vi "DB Info.vi"(8 "error in (no error)":errorcluster, 11 "Access in":refnum<class "Access.lvclass">) -> (0 "error out":errorcluster, 1 "Column_info":T1, 2 "Table_info":T4, 3 "Access out":refnum<class "Access.lvclass">)   [LabVIEW 2021, in "Database.lvlib" / "Access.lvclass"]
uses:
  Access.lvclass
  DB/Table_info.ctl
  DB/Column_info.ctl
  <vilib>/addons/database/Auxilliary.llb/DB Tools Column Info.ctl
  <vilib>/addons/database/Auxilliary.llb/DB Tools DataTypes.ctl
  DB/DB.lvclass
  <vilib>/addons/database/NI_Database_API.lvlib
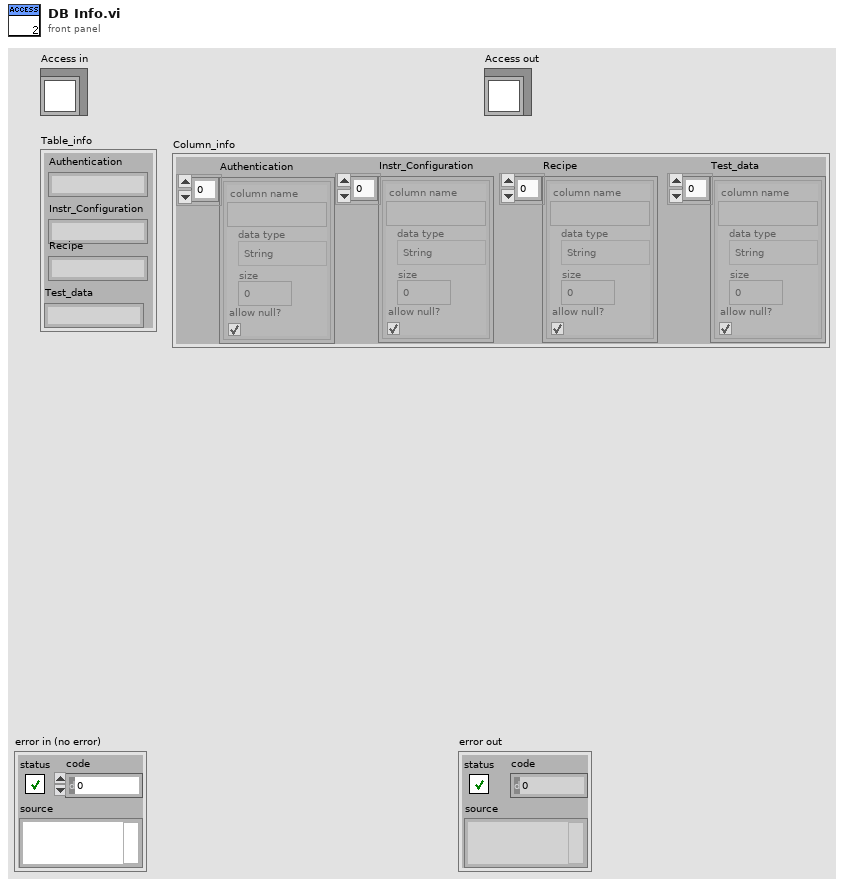
[diagram p1: front panel]
types:
  T1 = typedef "Database.lvlib/DB.lvclass/Column_info.ctl" = cluster{"Authentication":T2[], "Instr_Configuration":T2[], "Recipe":T2[], "Test_data":T2[]}
  T2 = typedef "NI_Database_API.lvlib/DB Tools Column Info.ctl" = cluster{"column name":string, "data type":T3, "size":i32, "allow null?":bool}
  T3 = typedef "NI_Database_API.lvlib/DB Tools DataTypes.ctl" = enum16{"String", "Long (I32)", "Single (SGL)", "Double (DBL)", "Date/Time", "Binary"}
  T4 = typedef "Database.lvlib/DB.lvclass/Table_info.ctl" = cluster{"Authentication":string, "Instr_Configuration":string, "Recipe":string, "Test_data":string}
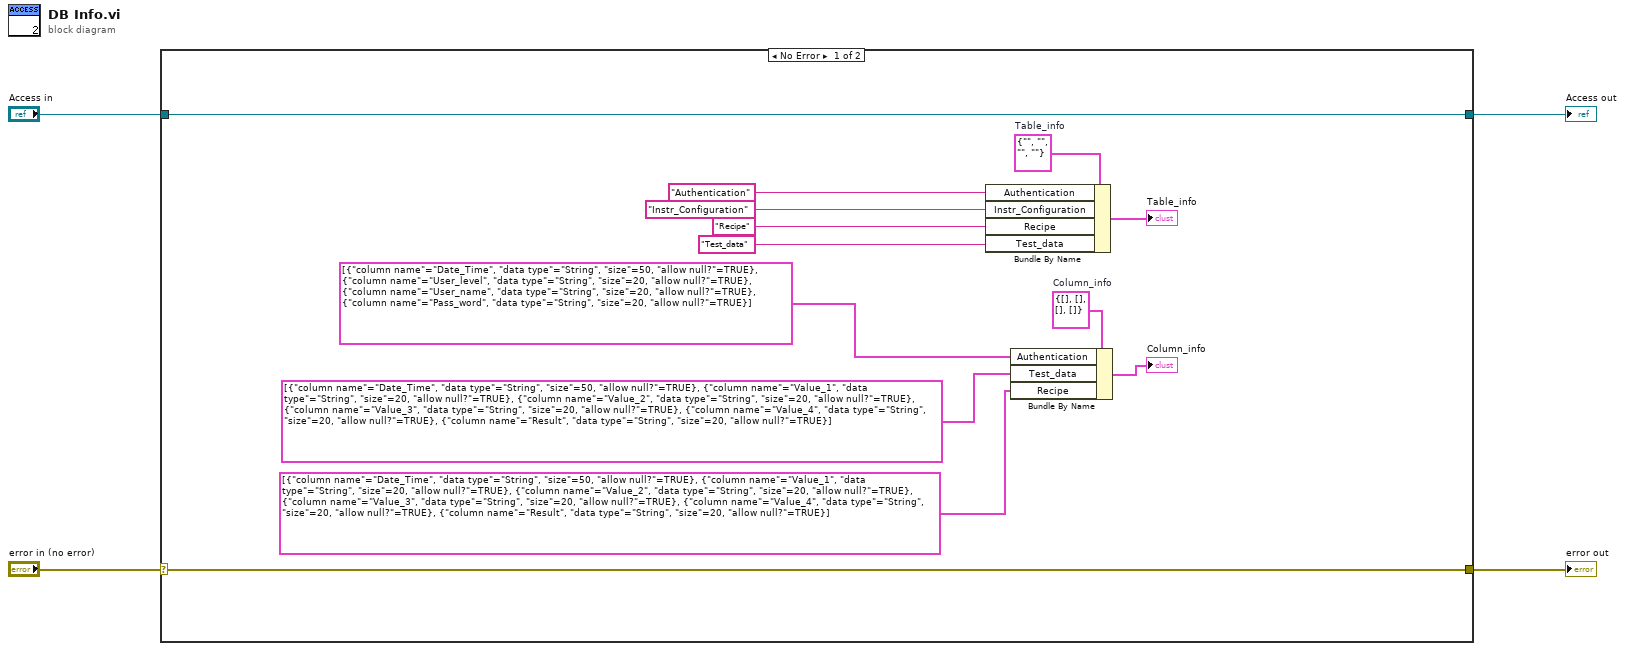
[diagram p0: block diagram]
diagram:
  n1 = case shown="No Error" "error in (no error)" {
    selector: "error in (no error)" -> [w17 w18]
    tunnel: "Access in" -> [w16 w19]
    tunnel: [w17 w18] -> w2
    tunnel: [w16 w19] -> w1
    frame No Error {
      w9 = T1 {"Authentication"=[], "Instr_Configuration"=[], "Recipe"=[], "Test_data"=[]}  # Column_info
      w15 = T4 {"Authentication"="", "Instr_Configuration"="", "Recipe"="", "Test_data"=""}  # Table_info
      n2 = Bundle By Name(cluster=w15, "Authentication"="Authentication", "Instr_Configuration"="Instr_Configuration" ("Table_2"), "Recipe"="Recipe" ("Table_3"), "Test_data"="Test_data" ("Table_4")) -> (→"Table_info":T4)
      n3 = Bundle By Name(cluster=w9, "Authentication"=T2[] [{"column name"="Date_Time", "data type"=enum."String", "size"=50, "allow null?"=TRUE}, {"column name"="User_level", "data type"=enum."String", "size"=20, "allow null?"=TRUE}, {"column name"="User_name", "data type"=enum."String", "size"=20, "allow null?"=TRUE}, {"column name"="Pass_word", "data type"=enum."String", "size"=20, "allow null?"=TRUE}], "Test_data"=T2[] [{"column name"="Date_Time", "data type"=enum."String", "size"=50, "allow null?"=TRUE}, {"column name"="Value_1", "data type"=enum."String", "size"=20, "allow null?"=TRUE}, {"column name"="Value_2", "data type"=enum."String", "size"=20, "allow null?"=TRUE}, {"column name"="Value_3", "data type"=enum."String", "size"=20, "allow null?"=TRUE}, {"column name"="Value_4", "data type"=enum."String", "size"=20, "allow null?"=TRUE}, {"column name"="Result", "data type"=enum."String", "size"=20, "allow null?"=TRUE}] ("Authentication"), "Recipe"=T2[] [{"column name"="Date_Time", "data type"=enum."String", "size"=50, "allow null?"=TRUE}, {"column name"="Value_1", "data type"=enum."String", "size"=20, "allow null?"=TRUE}, {"column name"="Value_2", "data type"=enum."String", "size"=20, "allow null?"=TRUE}, {"column name"="Value_3", "data type"=enum."String", "size"=20, "allow null?"=TRUE}, {"column name"="Value_4", "data type"=enum."String", "size"=20, "allow null?"=TRUE}, {"column name"="Result", "data type"=enum."String", "size"=20, "allow null?"=TRUE}] ("Authentication")) -> (→"Column_info":T1)
    }
    frame Error {
    }
  }
  "error out" <- w2
  "Access out" <- w1
